vi "cases_selector.vi"(0 "Q - quantidade (p.u.)":string, 1 "N - nó":string, 2 "C - condição de carga (p.u.)":string, 3 "Z - impedância de falta (Ohms)":string, 4 "I - instante de falta (ms)":string, 5 "L - local de falta":string, 6 "E - evento":string, 7 "T - tipo de falta":string, 8 "Parâmetros":string[](array[string])=["E", "Q", "N", "C", "Z", "M", "I", "L", "T", "M"], 9 "M - mecânica":string) -> (15 "nome do arquivo":string, 18 "dados":string[](array[string]))   [LabVIEW 2020]
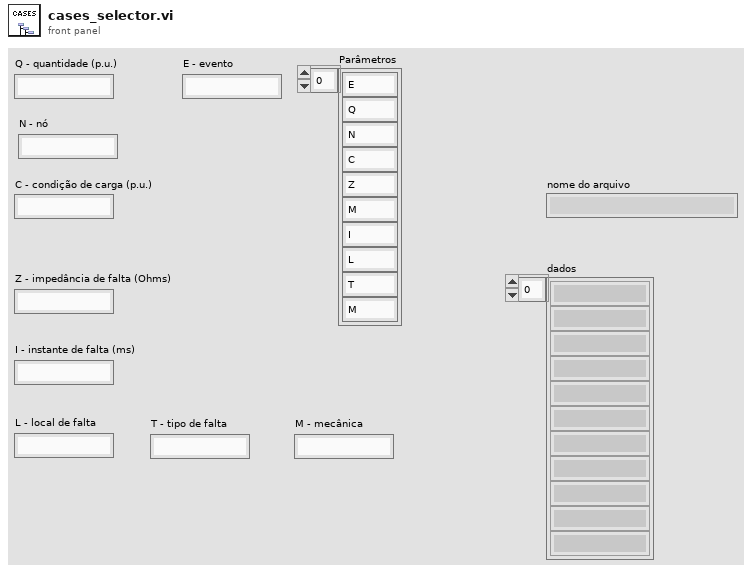
[diagram p1: front panel]
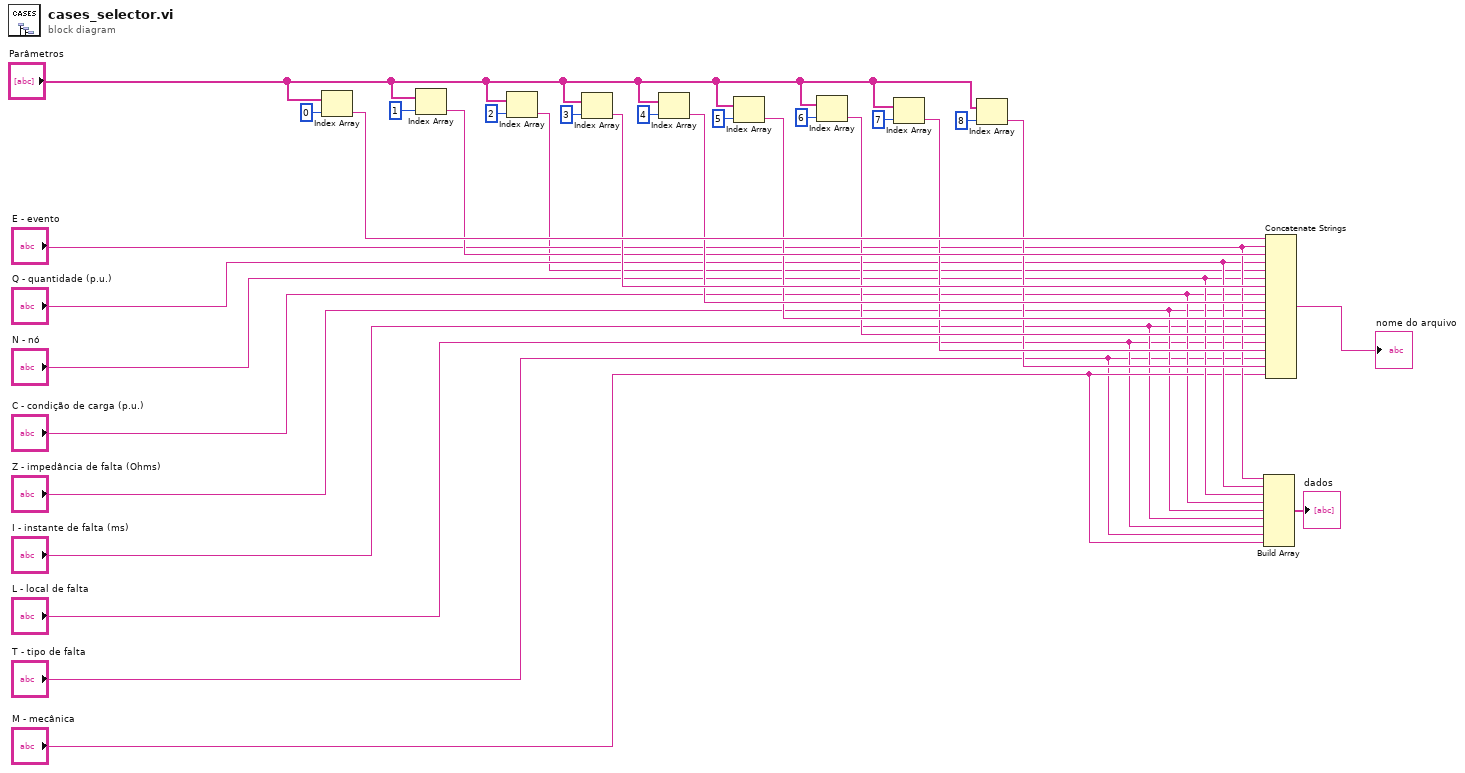
[diagram p0: block diagram]
diagram:
  n1 = Index Array(array="Parâmetros", index=0) -> (element=w28:string)
  n2 = Index Array(array="Parâmetros", index=1) -> (element=w22:string)
  n3 = Index Array(array="Parâmetros", index=2) -> (element=w9:string)
  n4 = Index Array(array="Parâmetros", index=3) -> (element=w24:string)
  n5 = Index Array(array="Parâmetros", index=4) -> (element=w23:string)
  n6 = Index Array(array="Parâmetros", index=5) -> (element=w20:string)
  n7 = Index Array(array="Parâmetros", index=6) -> (element=w18:string)
  n8 = Index Array(array="Parâmetros", index=7) -> (element=w14:string)
  n9 = Index Array(array="Parâmetros", index=8) -> (element=w13:string)
  n10 = Build Array("E - evento", "Q - quantidade (p.u.)", "N - nó", "C - condição de carga (p.u.)", "Z - impedância de falta (Ohms)", "I - instante de falta (ms)", "L - local de falta", "T - tipo de falta", "M - mecânica") -> (→"dados":string[])
  n11 = Concatenate Strings(w28, "E - evento", w22, "Q - quantidade (p.u.)", w9, "N - nó", w24, "C - condição de carga (p.u.)", w23, "Z - impedância de falta (Ohms)", w20, "I - instante de falta (ms)", w18, "L - local de falta", w14, "T - tipo de falta", w13, "M - mecânica") -> (→"nome do arquivo":string)
